vi "Set user event Show_HMI.vi"(8 "error in (no error)":errorcluster caption="entrée d'erreur (pas d'erreur)", 10 "user event Show_HMI":refnum<user-event>, 11 "Actor_Log en entrée":refnum<class "Actor_Log.lvclass">) -> (0 "error out":errorcluster caption="sortie d'erreur", 3 "Actor_Log en sortie":refnum<class "Actor_Log.lvclass">)   [LabVIEW 2020, in "Library Core.lvlib" / "Actor_Log.lvlib" / "Actor_Log.lvclass"]
uses:
  Actor_Log.lvclass
  Actor_Log.lvclass/Actor_Log.ctl
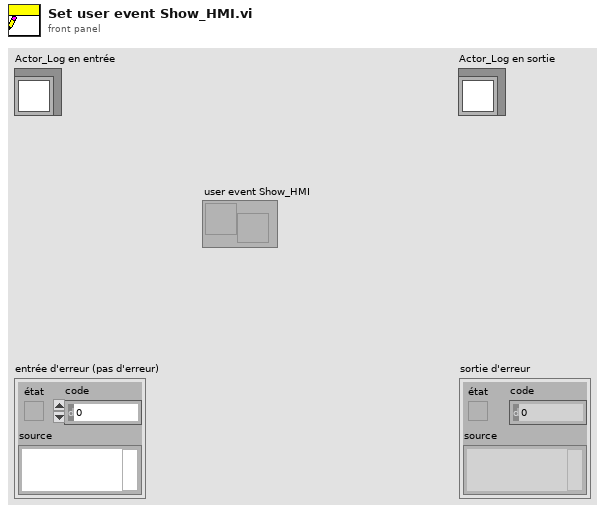
[diagram p1: front panel]
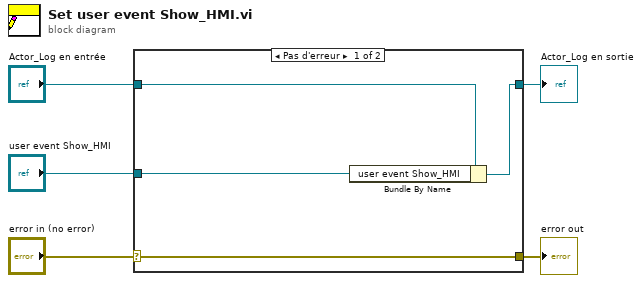
[diagram p0: block diagram]
diagram:
  n1 = case shown="Pas d'erreur" "error in (no error)" {
    selector: "error in (no error)" -> [w9 w10]
    tunnel: [w9 w10] -> w4
    tunnel: [w7 w11] -> w2
    tunnel: "Actor_Log en entrée" -> [w8 w11]
    tunnel: "user event Show_HMI" -> [w6 _]
    frame No Error {
      n2 = Bundle By Name(cluster=w8, "user event Show_HMI"=w6) -> (w7:refnum<class "Actor_Log.lvclass">)
    }
    frame Error {
    }
  }
  "error out" <- w4
  "Actor_Log en sortie" <- w2
